vi "Units to string.vi"(11 "Units":T1) -> (3 "Peak app":string)   [LabVIEW 2019, in "STAV lib.lvlib"]
uses:
  STAV lib.lvlib
  Param Units.ctl
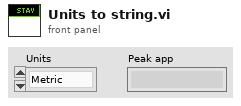
[diagram p1: front panel]
types:
  T1 = typedef "STAV lib.lvlib/Param Units.ctl" = enum16{"Metric", "Imperial"}
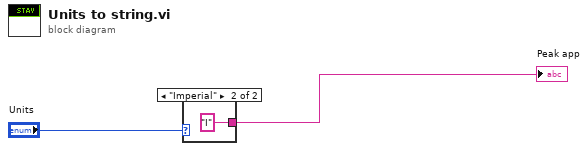
[diagram p0: block diagram]
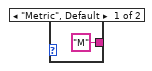
[diagram p2: hidden frame]
diagram:
  n1 = case shown="\"Imperial\"" "Units" {
    tunnel: ["M" ("Peak app") "I" ("Peak app")] -> w2
    frame "Metric", Default {
    }
    frame "Imperial" {
    }
  }
  "Peak app" <- w2
